vi "Serial_Logging_Global.vi"() -> ()   [LabVIEW 2018]
uses:
  Port_Params.ctl
panel:
  out "Port Settings Array":T1[](array[typedef]) {"flow control etc."."parity err byte" format="%.0x"; "flow control etc."."XON byte" format="%.0x"; "flow control etc."."XOFF byte" format="%.0x"; "data bits" min=5 max=8 step=1}
  in  "Commands to log (Default All)":string[](array[string])
  in  "Log Array3":string[](array[string])
  in  "Log Array2":string[](array[string])
  in  "Log Array1":string[](array[string])
  in  "Channels to Log":string[](array[string])
  in  "Serial Logging":bool
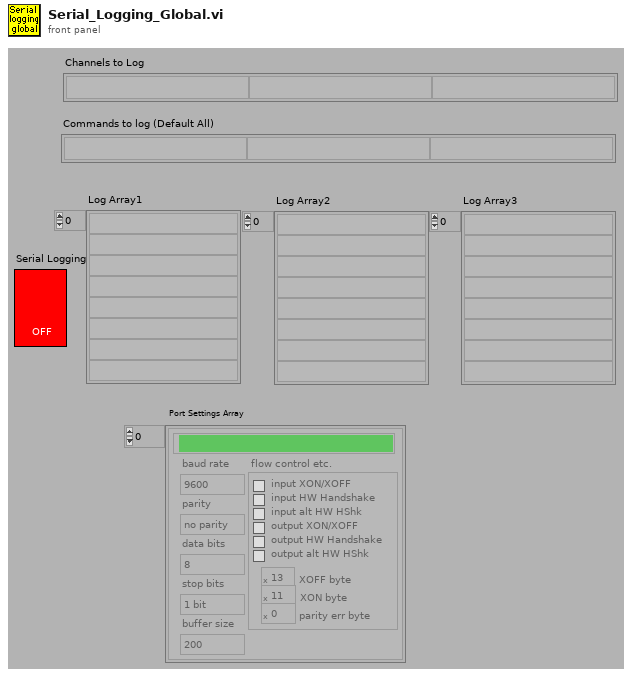
[diagram p1: front panel]
types:
  T1 = typedef "Port_Params.ctl" = cluster{"Name":string, "flow control etc.":cluster{"input XON/XOFF":bool, "input HW Handshake":bool, "input alt HW HShk":bool, "output XON/XOFF":bool, "output HW Handshake":bool, "output alt HW HShk":bool, "XOFF byte ":u8, "XON byte":u8, "parity err byte":u16}, "buffer size":u16, "baud rate":u32, "data bits":u16, "stop bits":enum16{"1 bit", "1.5 bits", "2 bits"}, "parity":enum16{"no parity", "odd parity", "even parity", "mark parity", "space parity"}}
diagram:
